vi "LiftControl.vi"(8 "error in (no error)":errorcluster, 9 "Autonomous?":bool=TRUE, 10 "LiftLevel Auto?":i32=3, 11 "Lift in":refnum<class "Lift.lvclass">) -> (0 "error out":errorcluster, 3 "Lift out":refnum<class "Lift.lvclass">)   [LabVIEW 2018, in "Lift.lvclass"]
uses:
  Lift.lvclass
  Lift.lvclass/Lift.ctl
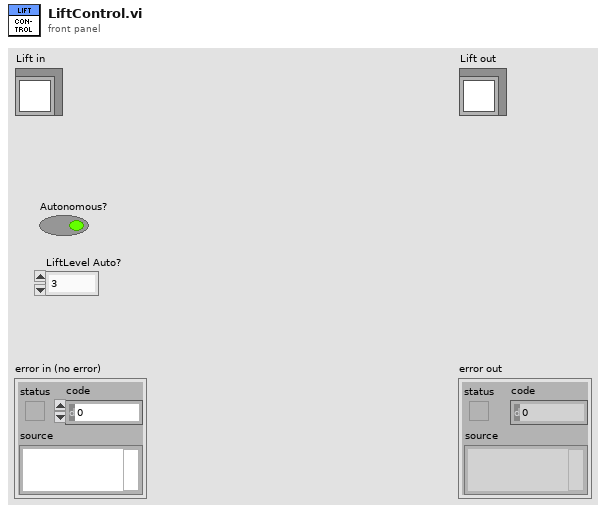
[diagram p1: front panel]
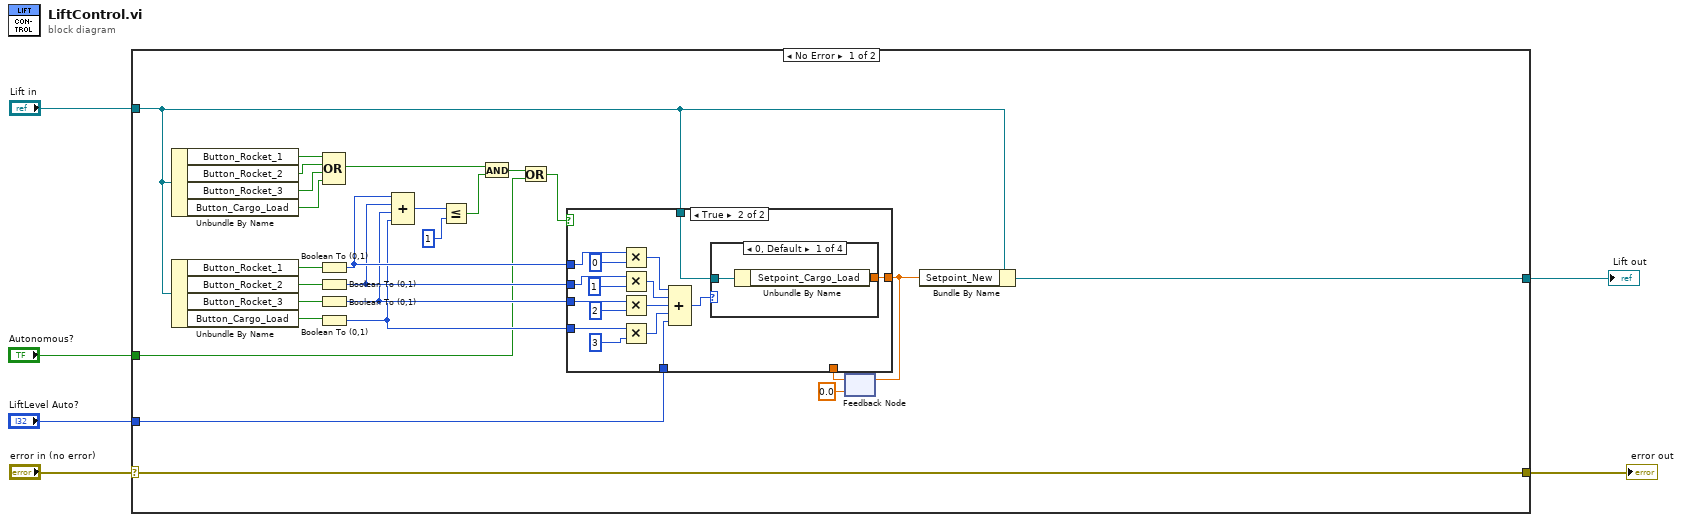
[diagram p0: block diagram]
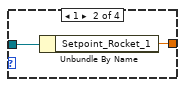
[diagram p3: hidden frame]
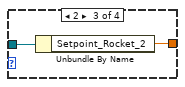
[diagram p4: hidden frame]
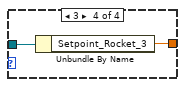
[diagram p5: hidden frame]
diagram:
  n1 = case shown="No Error" "error in (no error)" {
    selector: "error in (no error)" -> [w32 w59]
    tunnel: [w32 w59] -> w5
    tunnel: "Lift in" -> [w10 w58]
    tunnel: [w9 w58] -> w3
    tunnel: "Autonomous?" -> [w8 _]
    tunnel: "LiftLevel Auto?" -> [w7 _]
    frame No Error {
      n2 = Unbundle By Name(w10) -> ("Button_Rocket_1"=w31:bool, "Button_Rocket_2"=w30:bool, "Button_Rocket_3"=w29:bool, "Button_Cargo_Load"=w15:bool)
      n3 = Unbundle By Name(w10) -> ("Button_Rocket_1"=w28:bool, "Button_Rocket_2"=w27:bool, "Button_Rocket_3"=w26:bool, "Button_Cargo_Load"=w14:bool)
      n4 = Boolean To (0,1)(Boolean=w28) -> (0, 1=w21:i16)
      n5 = Boolean To (0,1)(Boolean=w27) -> (0, 1=w20:i16)
      n6 = Boolean To (0,1)(Boolean=w26) -> (0, 1=w19:i16)
      n7 = Boolean To (0,1)(Boolean=w14) -> (0, 1=w13:i16)
      n8 = Compound Arithmetic op=OR(w31, w30, w29, w15) -> (w22:bool)
      n9 = Compound Arithmetic op=ADD(w21, w20, w19, w13) -> (w24:i16)
      n10 = Less Or Equal?(x=w24, y=i16 1) -> (x <= y?=w23:bool)
      n11 = And(x=w22, y=w23) -> (x .and. y?=w12:bool)
      n12 = Or(x=w12, y=w8) -> (x .or. y?=w11:bool)
      n13 = feedback #1(0.0 ("Setpoint_High")) -> (w18:dbl)
      n14 = case shown="True" w11 {
        tunnel: w19 -> [_ w45]
        tunnel: w20 -> [_ w43]
        tunnel: w21 -> [_ w41]
        tunnel: [w33 w39] -> w16
        tunnel: w10 -> [_ w38]
        tunnel: w18 -> [w33 _]
        tunnel: w13 -> [_ w37]
        tunnel: w7 -> [_ w34]
        frame False {
        }
        frame True {
          n15 = Multiply(x=w41, y=0) -> (x*y=w47:i32)
          n16 = Multiply(x=w43, y=1) -> (x*y=w49:i32)
          n17 = Multiply(x=w45, y=2) -> (x*y=w48:i32)
          n18 = Multiply(x=w37, y=3) -> (x*y=w35:i32)
          n19 = Compound Arithmetic op=ADD(w47, w49, w48, w35, w34) -> (w40:i32)
          n20 = case shown="0, Default" w40 {
            tunnel: [w50 w52 w54 w56] -> w39
            tunnel: w38 -> [w51 w53 w55 w57]
            frame 0, Default {
              n21 = Unbundle By Name(w51) -> ("Setpoint_Cargo_Load"=w50:dbl)
            }
            frame 1 {
              n22 = Unbundle By Name(w53) -> ("Setpoint_Rocket_1"=w52:dbl)
            }
            frame 2 {
              n23 = Unbundle By Name(w55) -> ("Setpoint_Rocket_2"=w54:dbl)
            }
            frame 3 {
              n24 = Unbundle By Name(w57) -> ("Setpoint_Rocket_3"=w56:dbl)
            }
          }
        }
      }
      n25 = feedback-in #1(w16) -> ()
      n26 = Bundle By Name(cluster=w10, "Setpoint_New"=w16) -> (w9:refnum<class "Lift.lvclass">)
    }
    frame Error {
    }
  }
  "error out" <- w5
  "Lift out" <- w3
